vi "Sequence step namer.vi"(1 "number":i32) -> (0 "Step name":string)   [LabVIEW 2011]
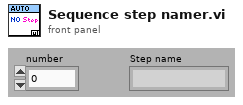
[diagram p1: front panel]
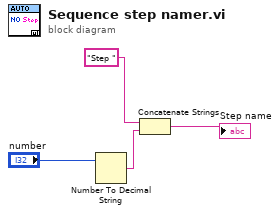
[diagram p0: block diagram]
diagram:
  n1 = Number To Decimal String(number="number") -> (decimal integer string=w2:string)  [unwired: 1 in]
  n2 = Concatenate Strings("Step " ("Section(Default)"), w2) -> (→"Step name":string)
